vi "LIDAR V7 FPGA Main.vi"() -> ()   [LabVIEW 2013]
uses:
  Controls/FPGA Nain State.ctl
  Controls/Scan Format Typedaf.ctl
  <vilib>/Platform/TimedLoop/XDataNode/timing_clust.ctl
  <vilib>/Platform/TimedLoop/XDataNode/nitl_modes.ctl
  <vilib>/Platform/TimedLoop/XDataNode/wakeup.ctl
  Controls/Algorithm State.ctl
  <vilib>/rvi/Emulation/niFpgaSctlEmulationGetInTimedLoop.vi
  <vilib>/rvi/Emulation/niFpgaEmulationReportErrorSimple.vi
  <vilib>/rvi/Emulation/niFpgaGetClockAttributes.vi
  <vilib>/rvi/FIFO/Fifo_Resource/nirvififoEmulationReadFpgaImpl.vi
  <vilib>/rvi/DataTransferAndStorage/Container/Common/niFpgaContainerGetUniqueNameForEmu.vi
  <vilib>/rvi/eio/common/nirviEmuTemplateMethod_errors.vi
  <vilib>/rvi/Emulation/niFpgaCriticalErrorInLSC.vi
  <vilib>/rvi/Emulation/niFpgaProcessEmulError.vi
  LIDAR V2 Globals.vi
  <vilib>/rvi/FIFO/Fifo_Resource/nirvififoEmulationWriteFpgaImpl.vi
  <vilib>/rvi/IPIntegrationNode/IPINode_Utilities/niFpgaIPINodeSimCore.vi
  <vilib>/rvi/interface/RandomDataEmulation/nirviRandomDataFPGAFIFO.vi
  <vilib>/rvi/interface/RandomDataEmulation/niFpgaRandomDataHandleErrors.vi
  <vilib>/Platform/TimedLoop/XDataNode/XDataNode.xnode
  <vilib>/rvi/DataTransferAndStorage/Container/XNode/niFpgaContainer.xnode
  <vilib>/rvi/FIFO/Fifo_Resource/nirvififoEmulationRead.vi
  <vilib>/eio/EIONode/EIONode.xnode
  <vilib>/rvi/FIFO/Fifo_Resource/nirvififoEmulationWrite.vi
  <vilib>/rvi/XilinxIP/XIPIN_XNode/niFpgaXIPIN.xnode
  Frac Decimation test/FIR Compiler/FractionalDecimationV1.dll
  <vilib>/rvi/IPIntegrationNode/IPINode_Xnode/niFpgaIPINode.xnode
  <vilib>/rvi/FXPMathLib/FxpInterpret/XNode/nifxpmath_Interpret.xnode
  <vilib>/rvi/interface/RandomDataEmulation/nirviRandomDataFpgaReadWriteTemplate.vi
  <vilib>/Platform/TimedLoop/XDataNode/XDNodeRunTimeDep.lvlib
panel:
  out "AI 0":i16
  in  "MaxStartSample":u8
  in  "LedScanDebEn":bool
  in  "ActiveLedIndexDeb":u16
  in  "10thIndexDeb":u8
  in  "PulseUpClck":u16=3
  in  "PulseWaitClck":u16=40
  in  "AO Trig":bool
  in  "Devider":u8=3
  in  "PFI3":bool
  in  "PFI2":bool
  in  "User Command Commit":bool
  in  "User Command":u8
  out "User Command Idle":bool
  out "User Command Status":u8
  in  "User Data 0":u8
  in  "User Data 1":u8
  out "User Error":bool
  out "Configured?":bool
  in  "MemDebStart":u32
  in  "MemDebEnd":u32
  in  "ReadMemSel":bool
  in  "ReadMem":bool
  in  "NextLedEn":bool
  out "SimCoarsMaxIndex":u16
  out "SimFineMaxIndex":u16
  out "SimOut":i16
  out "SPI Idle":bool
  out "PLL Locked":bool
  in  "Clock":u8=1
  out "PLL Counter":i32
  in  "IO Module\\Apply Settings":bool
  out "LedAddress":u16
  in  "SingleCycle":bool
  in  "PulsePerLed":i16=199
  in  "ScanFormat":T1=enum."FullScanPerLed"
  in  "SamplingEnable":bool
  out "MainState":T2
  out "10thIndex":u8
  out "PulseIndex":i16
  in  "MemSel":bool
  in  "ActiveLedIndex":u16
  out "InitMem":bool
  out "PulseEnd":bool
  in  "SampPerPulse":u16=99
  out "IterReset":u16 format="%.0b"
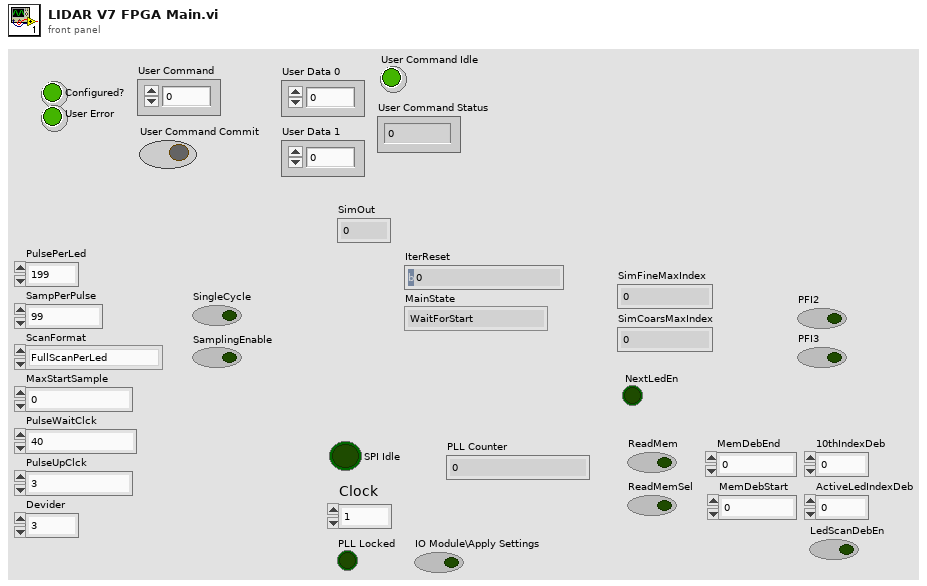
[diagram p1: front panel]
types:
  T1 = typedef "Scan Format Typedaf.ctl" = enum16{"1PulsePerLed", "FullScanPerLed"}
  T2 = typedef "FPGA Nain State.ctl" = enum16{"WaitForStart", "SetProcParams", "SelectActiveLed", "ActivatePulse", "WaitForPulseEnd", "WaitForAlgoStart", "SingleCycleEnd"}
  T3 = typedef "XDNodeRunTimeDep.lvlib/timing_clust.ctl" = cluster{"Expected End [f-1]":u64, "Actual End [f-1]":u64, "Finished Late? [f-1]":bool, "Expected End [i-1]":u64, "Actual End [i-1]":u64, "Finished Late? [i-1]":bool, "Expected Start [i]":u64, "Actual Start [i]":u64, "Expected Start [f]":u64, "Actual Start [f]":u64, "Source Name":string, "Structure Name":string, "Period":i64, "Deadline":i64, "Offset":i64, "Start":i64, "Priority":i32, "Timeout":i32, "Mode":T4, "Wakeup Reason":T5, "Error":errorcluster, "Source Type":string, "Secondary Source Type":string, "Global End Time":u64, "Global Start Time":u64, "Frame Duration":u64, "Iteration Duration":u64, "Assigned CPU":i32, "I/O Scan Engine Mode":u32}
  T4 = typedef "XDNodeRunTimeDep.lvlib/nitl_modes.ctl" = enum32{"No Change", "Process missed periods, maintain original phase", "Discard missed periods, maintain original phase", "Process missed periods, ignore original phase", "Discard missed periods, ignore original phase"}
  T5 = typedef "XDNodeRunTimeDep.lvlib/wakeup.ctl" = enum32{"Normal", "Aborted", "Asynchronous wakeup", "Timing source error", "Timed loop error", "Timeout"}
  T6 = typedef "Algorithm State.ctl" = enum16{"WaitForStart", "GetNextSignalElement", "WaitForNextSignalElem", "MultWithSinc", "CalcMax"}
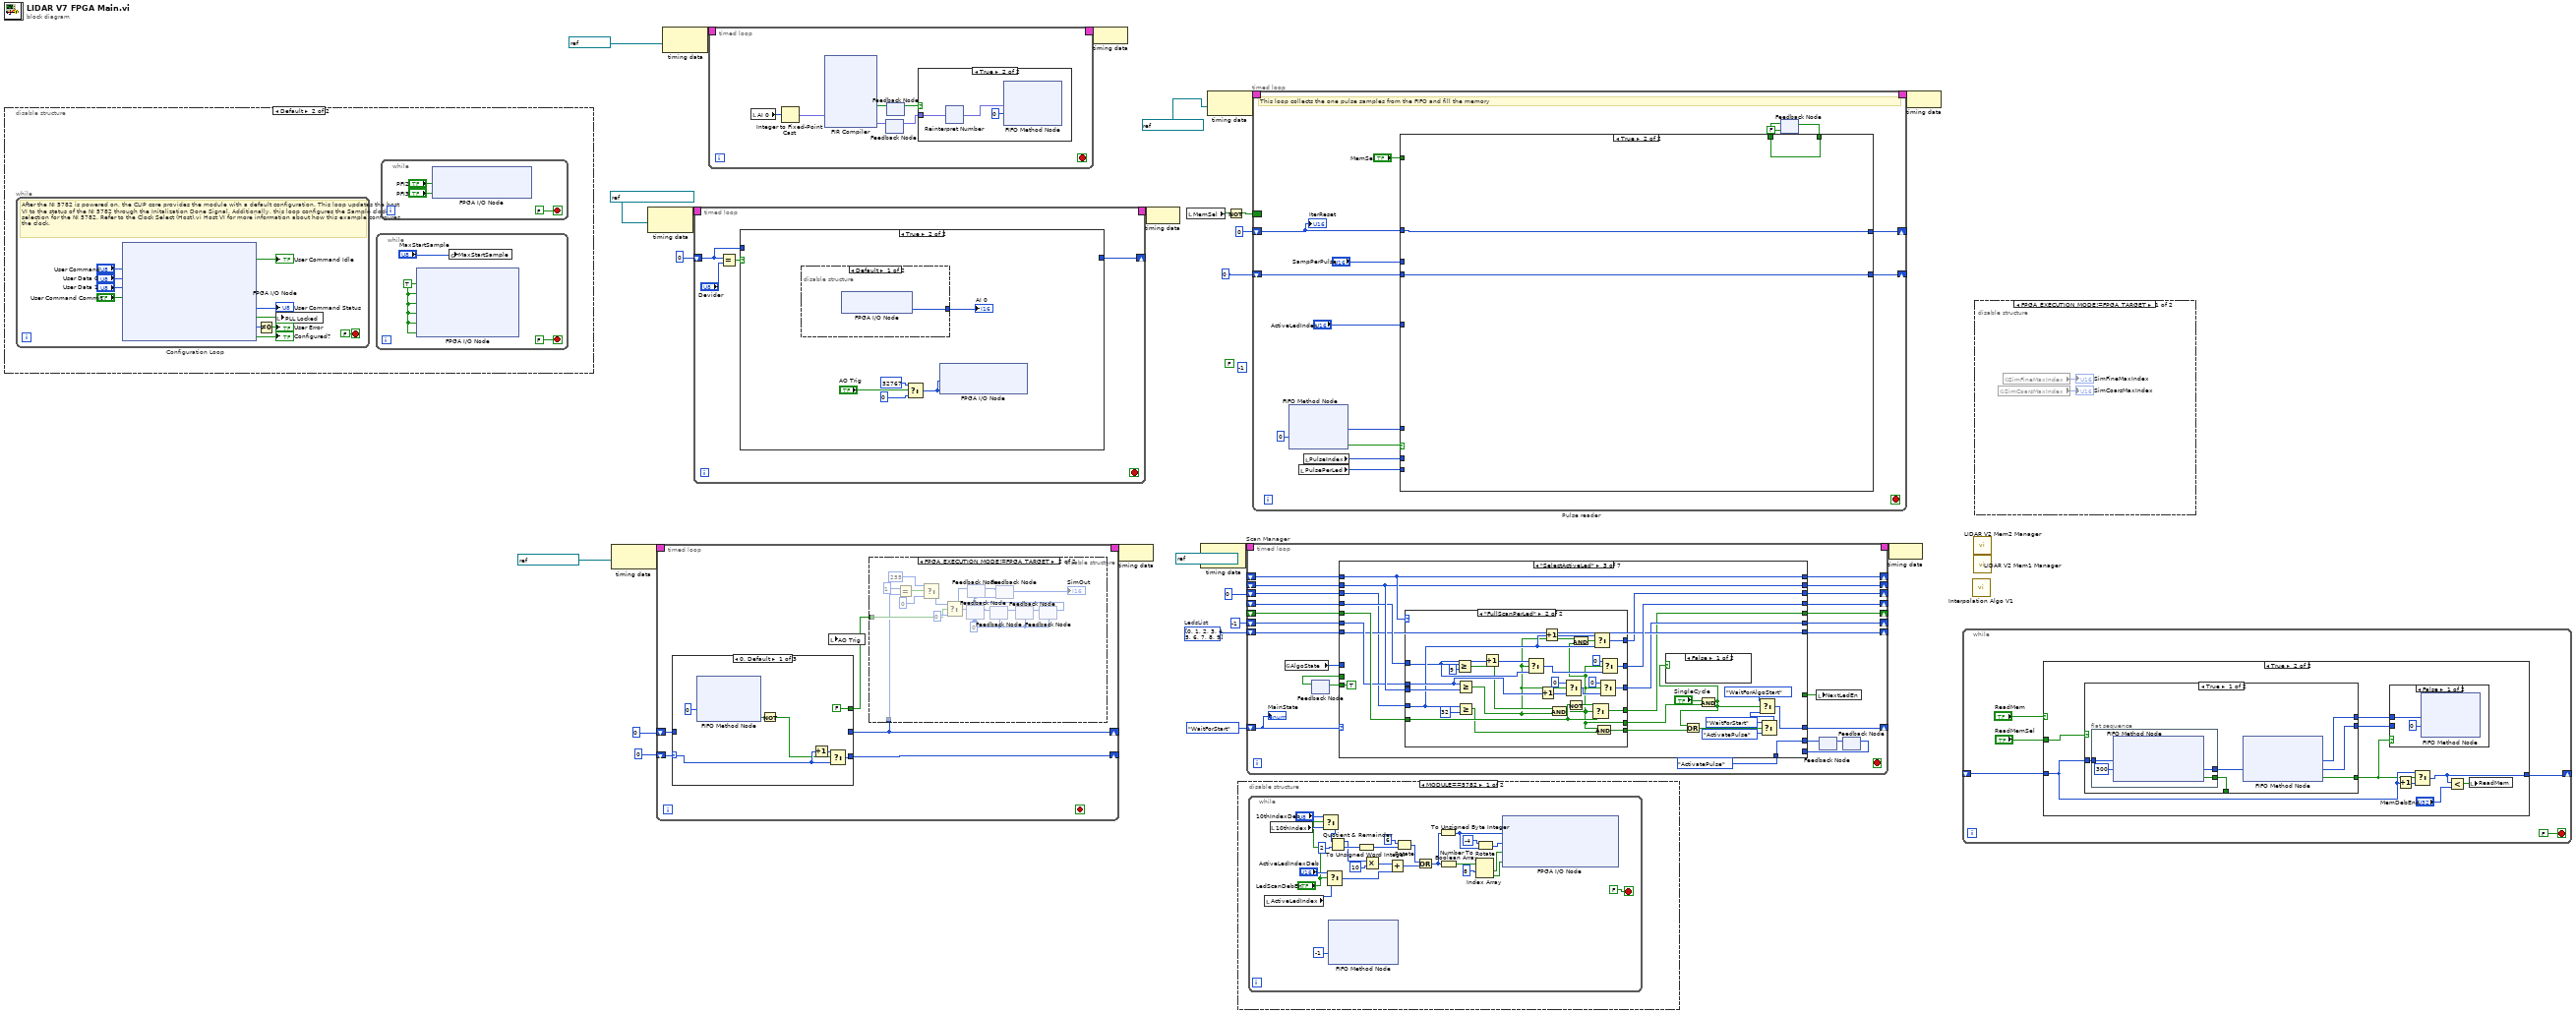
[diagram p0: block diagram]
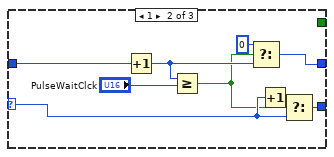
[diagram p4: hidden frame]
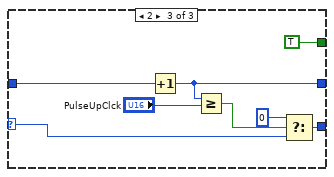
[diagram p5: hidden frame]
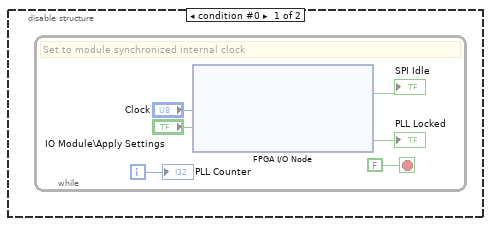
[diagram p7: hidden frame]
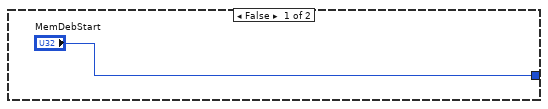
[diagram p8: hidden frame]
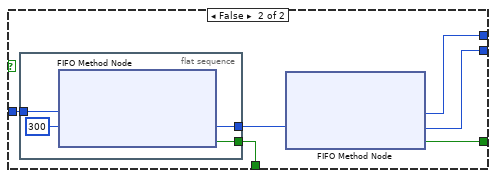
[diagram p10: hidden frame]
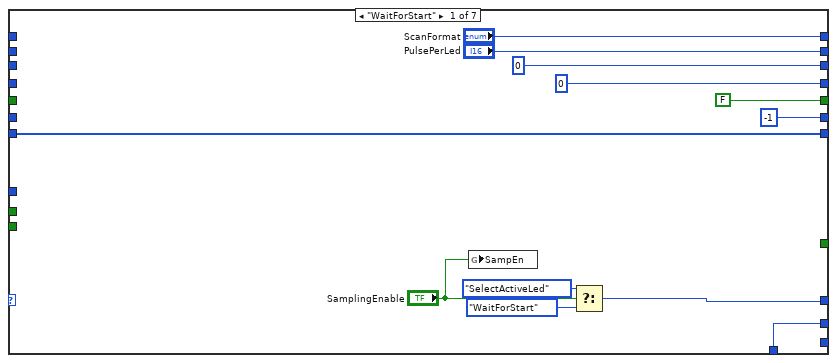
[diagram p12: hidden frame]
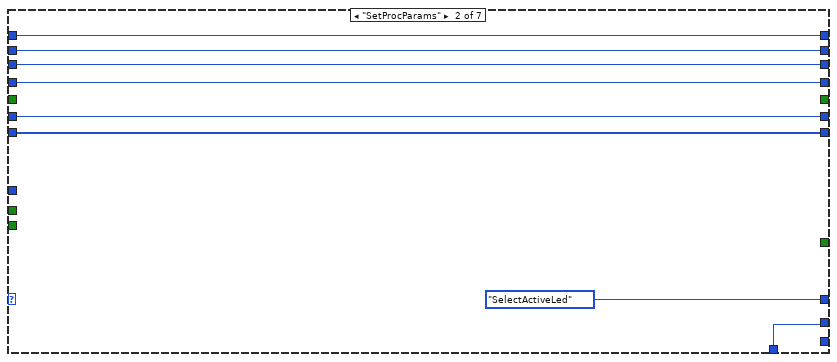
[diagram p13: hidden frame]
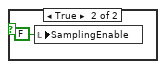
[diagram p14: hidden frame]
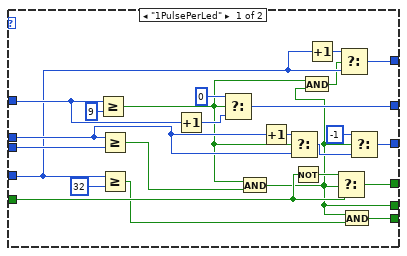
[diagram p15: hidden frame]
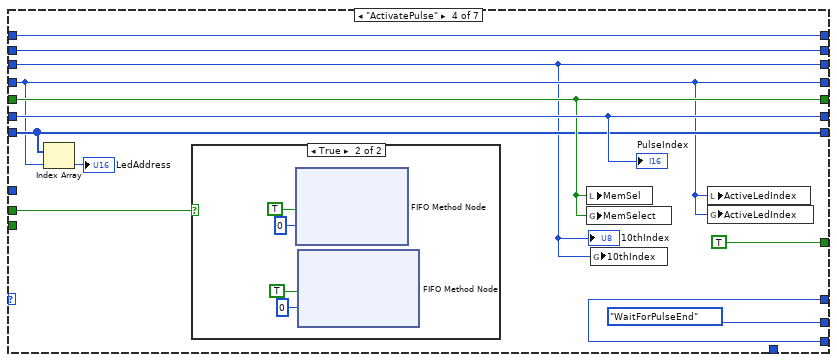
[diagram p16: hidden frame]
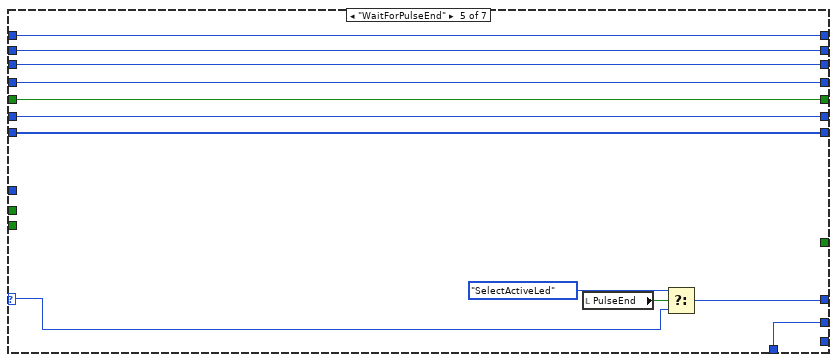
[diagram p18: hidden frame]
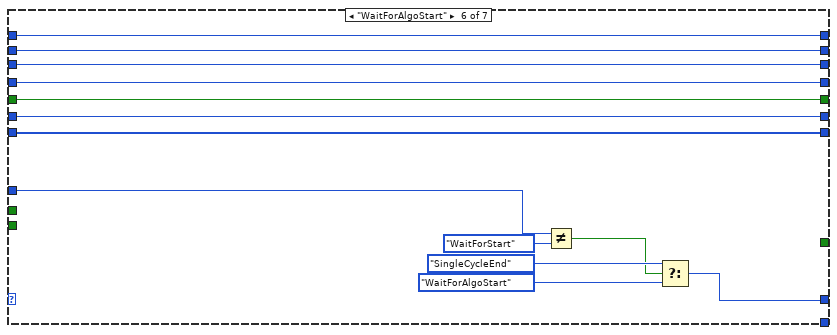
[diagram p19: hidden frame]
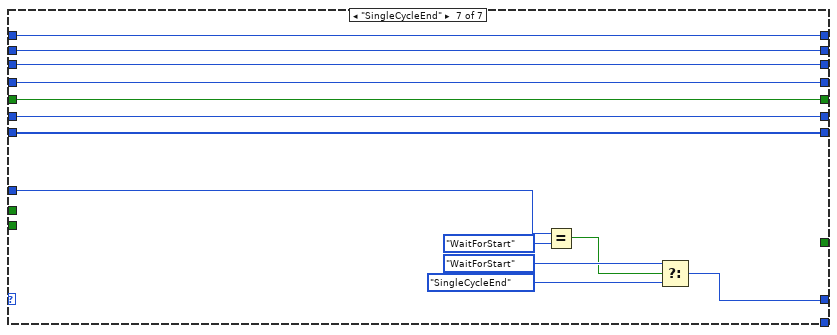
[diagram p20: hidden frame]
diagram:
  (unwired) FALSE
  w14 = u16[] [0, 1, 2, 3, 4, 5, 6, 7, 8, 9]  # LedsList
  (unwired) i16 -1 ("#Cycle")
  n1 = disable-structure shown="Default" {
    frame condition #0 {
      n2 = while {
        i -> [w29]
        stop <- FALSE stop-if-true
        # "Set to module synchronized internal clock"
        n3 = xnode "FPGA I/O Node"("IO Module\\Clock Select"="Clock", "IO Module\\Apply Settings"="IO Module\\Apply Settings") -> ("IO Module\\SPI Idle"=→"SPI Idle":bool, "IO Module\\PLL Locked"=→"PLL Locked":bool)  [unwired: 4 in, 4 out]
        "PLL Counter" <- w29
      }
    }
    frame condition #1 (active) {
      n4 = while "Configuration Loop" {
        stop <- FALSE stop-if-true
        # "After the NI 5782 is powered on, the CLIP core provides the module with a default configuration. This loop updates the host VI to the status of the NI 5782 through the Initalization Done Signal. Additionally, this loop configures the Sample clock selection for the NI 5782. Refer to the Clock Select (Host).vi Host VI for more information about how this example configures the clock."
        n5 = xnode "FPGA I/O Node"("IO Module\\User Command"="User Command", "IO Module\\User Data 0"="User Data 0", "IO Module\\User Data 1"="User Data 1", "IO Module\\User Command Commit"="User Command Commit") -> ("IO Module\\User Command Idle"=→"User Command Idle":bool, "IO Module\\User Command Status"=→"User Command Status":u8, "IO Module\\PLL Locked"=w36:bool, "IO Module\\User Error"=w40:u8, "IO Module\\Initialization Done"=→"Configured?":bool)  [unwired: 9 in, 9 out]
        n6 = Not Equal To 0?(x=w40) -> (x != 0?=→"User Error":bool)
        n7 = local write "PLL Locked"(w36) -> ()
      }
      n8 = while {
        stop <- FALSE stop-if-true
        w48 = TRUE ("IO Module\\DIO Port 0 WE")
        n9 = xnode "FPGA I/O Node"("IO Module\\DIO Port 0 WE"=w48, "IO Module\\DIO Port 1 WE"=w48, "IO Module\\PFI 0 WE"=w48, "IO Module\\PFI 1 WE"=w48, "IO Module\\PFI 2 WE"=w48, "IO Module\\PFI 3 WE"=w48) -> ()  [unwired: 6 in, 6 out]
        n10 = global write "LIDAR V2 Globals.vi" "MaxStartSample"("MaxStartSample") -> ()
      }
      n11 = while {
        stop <- FALSE stop-if-true
        n12 = xnode "FPGA I/O Node"("IO Module\\PFI 2 Wr Data"="PFI2", "IO Module\\PFI 3 Wr Data"="PFI3") -> ()  [unwired: 2 in, 2 out]
      }
    }
  }
  n13 = node-c288(refnum<k21> "100 MHz Clock" ("Source Name")) -> (w8:T3)
  n14 = node-c288(refnum<k21> "IO Module\\Data Clock" ("Source Name")) -> (w26:T3)
  n15 = timed-loop {
    timing: w8 -> [_]
    timing-out: [_] -> w7
    shift-right: [w53] -> _
    shift-left: i16 0 -> [w54]
    shift-right: [w51] -> _
    shift-left: u16 0 -> [w52]
    stop <- _ stop-if-true
    n16 = case shown="0, Default" w54 {
      selector: w54 -> [w76 w83 w89]
      tunnel: [w77 w84 w90] -> w53
      tunnel: w52 -> [_ w86 w94]
      tunnel: [_ w80 w93] -> w51
      tunnel: [FALSE _ TRUE] -> w50
      frame 0, Default {
        n17 = xnode ("FIFO Method Node")("Timeout"=0) -> ("Timed Out?"=w73:bool)  [unwired: 1 in, 2 out]
        n18 = Not(x=w73) -> (.not. x?=w71:bool)
        n19 = Increment(x=w76) -> (x+1=w75:i16)
        n20 = Select(t=w75, s=w71, f=w76) -> (s? t:f=w77:i16)
      }
      frame 1 {
        n21 = Increment(x=w86) -> (x+1=w81:u16)
        n22 = Greater Or Equal?(x=w81, y="PulseWaitClck") -> (x >= y?=w78:bool)
        n23 = Select(t=u16 0, s=w78, f=w81) -> (s? t:f=w80:u16)
        n24 = Increment(x=w83) -> (x+1=w82:i16)
        n25 = Select(t=w82, s=w78, f=w83) -> (s? t:f=w84:i16)
      }
      frame 2 {
        n26 = Increment(x=w94) -> (x+1=w93:u16)
        n27 = Greater Or Equal?(x=w93, y="PulseUpClck") -> (x >= y?=w91:bool)
        n28 = Select(t=i16 0, s=w91, f=w89) -> (s? t:f=w90:i16)
      }
    }
    n29 = local write "AO Trig"(w50) -> ()
    n30 = disable-structure shown="FPGA_EXECUTION_MODE!=FPGA_TARGET" {
      disable-tunnel: w50 -> [_ w62]
      disable-tunnel: w51 -> [_ w61]
      frame condition #0 (active) {
      }
      frame condition #1 {
        w65 = i16 0 ("IO Module\\AO 0")
        n31 = Equal?(x=u16 1, y=w61) -> (x = y?=w59:bool)
        n32 = Select(t=i16 255 ("IO Module\\AO 0"), s=w59, f=i16 0) -> (s? t:f=w60:i16)
        n33 = Select(t=w60, s=w62, f=i16 0 ("IO Module\\AO 0")) -> (s? t:f=w63:i16)
        n34 = feedback-in #1(w63) -> ()
        n35 = feedback #1(w65) -> (w70:i16)
        n36 = feedback #2(w65) -> (w66:i16)
        n37 = feedback #3(w65) -> (w69:i16)
        n38 = feedback-in #3(w70) -> ()
        n39 = feedback #4(w65) -> (→"SimOut":i16)
        n40 = feedback-in #4(w66) -> ()
        n41 = feedback #5(w65) -> (w68:i16)
        n42 = feedback-in #5(w69) -> ()
        n43 = feedback #6(w65) -> (w67:i16)
        n44 = feedback-in #2(w67) -> ()
        n45 = feedback-in #6(w68) -> ()
      }
    }
  }
  n46 = node-c288(refnum<k21> "300MHz" ("Source Name")) -> (w3:T3)
  n47 = timed-loop {
    timing: w26 -> [_]
    timing-out: [_] -> w25
    shift-right: [w97] -> _
    shift-left: u8 0 -> [w98]
    stop <- _ stop-if-true
    n48 = Equal?(x=w98, y="Devider") -> (x = y?=w99:bool)
    n49 = case shown="True" w99 {
      tunnel: w98 -> [w102 _]
      tunnel: [w101 _] -> w97
      frame False {
        n50 = Increment(x=w102) -> (x+1=w101:u8)
      }
      frame True {
        n51 = disable-structure shown="Default" {
          disable-tunnel: [w108 w109] -> w107
          frame condition #0 (active) {
            n52 = xnode "FPGA I/O Node"() -> ("IO Module\\AI 0"=w108:i16)  [unwired: 1 in, 1 out]
          }
          frame condition #1 {
            n53 = local read "SimOut"() -> (w109:i16)
          }
        }
        "AI 0" <- w107
        n54 = Select(t=i16 32767 ("IO Module\\AO 0"), s="AO Trig", f=i16 0 ("IO Module\\AO 0")) -> (s? t:f=w106:i16)
        n55 = xnode "FPGA I/O Node"("IO Module\\AO 0 N-1"=w106, "IO Module\\AO 0 N"=w106) -> ()  [unwired: 2 in, 2 out]
      }
    }
  }
  n56 = timed-loop {
    timing: w3 -> [_]
    timing-out: [_] -> w2
    stop <- _ stop-if-true
    n57 = local read "AI 0"() -> (w117:i16)
    n58 = Integer to Fixed-Point Cast(integer=w117) -> (fixed-point=w116:fxp<+/-,16,16>)  [unwired: 1 in]
    n59 = xnode ("FIR Compiler")("din"=w116) -> ("rdy"=w115:bool, "dout"=w114:fxp<+/-,33,33>)  [unwired: 1 out]
    n60 = feedback-in #7(w114) -> ()
    n61 = feedback #7() -> (w112:fxp<+/-,33,33>)  [unwired: 1 in]
    n62 = feedback-in #8(w115) -> ()
    n63 = feedback #8() -> (w113:bool)  [unwired: 1 in]
    n64 = case shown="True" w113 {
      tunnel: w112 -> [_ w166]
      frame False {
      }
      frame True {
        n65 = xnode "Reinterpret Number"("x"=w166) -> ("y"=w167:fxp<+/-,33,16>)
        n66 = xnode ("FIFO Method Node")("Element"=w167, "Timeout"=0) -> ()  [unwired: 1 in, 2 out]
      }
    }
  }
  n67 = node-c288(w2) -> ()
  n68 = node-c288(w7) -> ()
  n69 = node-c288(w25) -> ()
  n70 = local read "MemSel"() -> (w19:bool)
  n71 = node-c288(refnum<k21> "100 MHz Clock" ("Source Name")) -> (w22:T3)
  n72 = node-c288(refnum<k21> "100 MHz Clock" ("Source Name")) -> (w24:T3)
  n73 = Not(x=w19) -> (.not. x?=w18:bool)
  n74 = disable-structure shown="MODULE==5782" {
    frame condition #0 (active) {
      n75 = while {
        stop <- FALSE stop-if-true
        n76 = local read "ActiveLedIndex"() -> (w175:u16)
        n77 = local read "10thIndex"() -> (w177:u8)
        n78 = Select(t="10thIndexDeb", s="LedScanDebEn", f=w177) -> (s? t:f=w176:u8)
        n79 = Select(t="ActiveLedIndexDeb", s="LedScanDebEn", f=w175) -> (s? t:f=w174:u16)
        n80 = xnode ("FIFO Method Node")("Timeout"=-1) -> ()  [unwired: 1 in, 3 out]
        n81 = Quotient & Remainder(x=w176, y=u8 2) -> (x-y*floor(x/y)=w181:u8, floor(x/y)=w182:u8)
        n82 = To Unsigned Word Integer(number=w182) -> (unsigned 16bit integer=w189:u16)
        n83 = Multiply(x=w181, y=u8 10) -> (x*y=w180:u8)
        n84 = Add(x=w180, y=w174) -> (x+y=w195:u16)
        n85 = Rotate(1:w189, 2:u16 6 ("x")) -> (0:w196:u16)
        n86 = Or(x=w196, y=w195) -> (x .or. y?=w194:u16)
        n87 = To Unsigned Byte Integer(number=w194) -> (unsigned 8bit integer=w186:u8)
        n88 = Number To Boolean Array(number=w194) -> (Boolean array=w193:bool[])
        n89 = Index Array(array=w193, index #1=8 ("index")) -> (element #1=w191:bool, element #2=w190:bool)  [unwired: 1 in]
        n90 = Rotate(1:w186, 2:i16 -4 ("y")) -> (0:w184:u8)
        n91 = xnode "FPGA I/O Node"("IO Module\\DIO Port 0 Wr Data"=w186, "IO Module\\DIO Port 1 Wr Data"=w184, "IO Module\\PFI 0 Wr Data"=w191, "IO Module\\PFI 1 Wr Data"=w190) -> ()  [unwired: 4 in, 4 out]
      }
    }
    frame condition #1 {
    }
  }
  n92 = timed-loop "Scan Manager" {
    timing: w22 -> [_]
    timing-out: [_] -> w21
    shift-right: [w219] -> _
    shift-left: FPGA_Nain_State."WaitForStart" ("MainState") -> [w220]
    shift-right: [w218] -> _
    shift-left: _ -> [w216]
    shift-right: [w217] -> _
    shift-left: _ -> [w215]
    shift-right: [w208] -> _
    shift-left: u8 0 ("10thIndex") -> [w214]
    shift-right: [w198] -> _
    shift-left: _ -> [w213]
    shift-right: [w202] -> _
    shift-left: _ -> [w212]
    shift-right: [w211] -> _
    shift-left: i16 -1 -> [w201]
    shift-right: [w209] -> _
    shift-left: w14 -> [w210]
    stop <- _ stop-if-true
    n93 = global read "LIDAR V2 Globals.vi" "AlgoState"() -> (w197:T6)
    n94 = feedback #9() -> (w199:bool)  [unwired: 1 in]
    n95 = feedback #10() -> (w205:T2)  [unwired: 1 in]
    n96 = feedback #11() -> (w204:T2)  [unwired: 1 in]
    n97 = case shown="\"SelectActiveLed\"" w220 {
      selector: w220 -> [_ _ _ _ w336 _ _]
      tunnel: [w230 FPGA_Nain_State."SelectActiveLed" ("MainState") w244 w322 w335 w346 w359] -> w219
      tunnel: ["ScanFormat" w236 w263 w326 w342 w355 w368] -> w218
      tunnel: ["PulsePerLed" w235 w261 w325 w341 w354 w367] -> w217
      tunnel: w216 -> [_ w236 w263 w326 w342 w355 w368]
      tunnel: w215 -> [_ w235 w261 w325 w341 w354 w367]
      tunnel: [u8 0 ("10thIndex") w234 w252 w315 w340 w353 w366] -> w208
      tunnel: w214 -> [_ w234 w253 w315 w340 w353 w366]
      tunnel: [u16 0 ("ActiveLedIndex") w233 w258 w316 w339 w352 w365] -> w198
      tunnel: w213 -> [_ w233 w259 w316 w339 w352 w365]
      tunnel: [FALSE _ w255 w319 w338 w351 w364] -> w202
      tunnel: w212 -> [_ _ w262 w319 w338 w351 w364]
      tunnel: [i16 -1 ("t") w239 w256 w320 w333 w350 w363] -> w211
      tunnel: w201 -> [_ w239 w260 w320 w333 w350 w363]
      tunnel: w210 -> [w228 w238 w257 w317 w332 w349 w362]
      tunnel: [w228 w238 w257 w317 w332 w349 w362] -> w209
      tunnel: [_ _ _ TRUE ("SampEnable") _ _ _] -> w207
      tunnel: [w227 w237 w251 FPGA_Nain_State."WaitForPulseEnd" ("MainState") w331 _ _] -> w206
      tunnel: w204 -> [_ _ _ w322 _ _ _]
      tunnel: FPGA_Nain_State."ActivatePulse" ("MainState") -> [w227 w237 w251 _ w331 _ _]
      tunnel: [_ _ TRUE _ _ _ _] -> w200
      tunnel: w199 -> [_ _ _ w321 _ _ _]
      tunnel: w197 -> [_ _ _ _ _ w343 w357]
      frame "WaitForStart" {
        n98 = global write "LIDAR V2 Globals.vi" "SampEn"("SamplingEnable") -> ()
        n99 = Select(t=FPGA_Nain_State."SelectActiveLed" ("MainState"), s="SamplingEnable", f=FPGA_Nain_State."WaitForStart" ("MainState")) -> (s? t:f=w230:T2)
      }
      frame "SetProcParams" {
      }
      frame "SelectActiveLed" {
        n100 = case shown="\"FullScanPerLed\"" w263 {
          tunnel: w262 -> [w280 w310]
          tunnel: w253 -> [w273 w305]
          tunnel: w261 -> [w283 w312]
          tunnel: w259 -> [w286 w296]
          tunnel: w260 -> [w282 w311]
          tunnel: [w274 w292] -> w258
          tunnel: [w269 w294] -> w256
          tunnel: [w277 w308] -> w255
          tunnel: [w275 w306] -> w249
          tunnel: [w271 w303] -> w252
          tunnel: [w265 w289] -> w250
          frame "1PulsePerLed" {
            n101 = Greater Or Equal?(x=w286, y=u16 9) -> (x >= y?=w267:bool)
            n102 = Greater Or Equal?(x=w282, y=w283) -> (x >= y?=w278:bool)
            n103 = Greater Or Equal?(x=w273, y=u8 32) -> (x >= y?=w276:bool)
            n104 = Increment(x=w286) -> (x+1=w285:u16)
            n105 = Select(t=u16 0, s=w267, f=w285) -> (s? t:f=w274:u16)
            n106 = And(x=w267, y=w278) -> (x .and. y?=w265:bool)
            n107 = Increment(x=w282) -> (x+1=w281:i16)
            n108 = Select(t=w281, s=w267, f=w282) -> (s? t:f=w270:i16)
            n109 = Not(x=w280) -> (.not. x?=w279:bool)
            n110 = And(x=w267, y=w265) -> (x .and. y?=w266:bool)
            n111 = Increment(x=w273) -> (x+1=w272:u8)
            n112 = Select(t=w279, s=w265, f=w280) -> (s? t:f=w277:bool)
            n113 = Select(t=w272, s=w266, f=w273) -> (s? t:f=w271:u8)
            n114 = And(x=w265, y=w276) -> (x .and. y?=w275:bool)
            n115 = Select(t=i16 -1, s=w265, f=w270) -> (s? t:f=w269:i16)
          }
          frame "FullScanPerLed" {
            n116 = Greater Or Equal?(x=w296, y=u16 9) -> (x >= y?=w295:bool)
            n117 = Greater Or Equal?(x=w311, y=w312) -> (x >= y?=w290:bool)
            n118 = Greater Or Equal?(x=w305, y=u8 32) -> (x >= y?=w307:bool)
            n119 = Increment(x=w296) -> (x+1=w297:u16)
            n120 = Select(t=w297, s=w290, f=w296) -> (s? t:f=w293:u16)
            n121 = Increment(x=w311) -> (x+1=w299:i16)
            n122 = Increment(x=w305) -> (x+1=w304:u8)
            n123 = And(x=w295, y=w290) -> (x .and. y?=w289:bool)
            n124 = Select(t=i16 0, s=w290, f=w299) -> (s? t:f=w302:i16)
            n125 = Not(x=w310) -> (.not. x?=w309:bool)
            n126 = And(x=w290, y=w289) -> (x .and. y?=w300:bool)
            n127 = Select(t=w309, s=w289, f=w310) -> (s? t:f=w308:bool)
            n128 = Select(t=w304, s=w300, f=w305) -> (s? t:f=w303:u8)
            n129 = And(x=w289, y=w307) -> (x .and. y?=w306:bool)
            n130 = Select(t=i16 0, s=w289, f=w302) -> (s? t:f=w294:i16)
            n131 = Select(t=u16 0, s=w289, f=w293) -> (s? t:f=w292:u16)
          }
        }
        n132 = And(x="SingleCycle", y=w250) -> (x .and. y?=w241:bool)
        n133 = case shown="False" w241 {
          frame False {
          }
          frame True {
            n134 = local write "SamplingEnable"(FALSE ("SamplingEnable")) -> ()
          }
        }
        n135 = Or(x=w241, y=w249) -> (x .or. y?=w248:bool)
        n136 = Select(t=FPGA_Nain_State."WaitForStart" ("MainState"), s=w248, f=FPGA_Nain_State."ActivatePulse" ("MainState")) -> (s? t:f=w245:T2)
        n137 = Select(t=FPGA_Nain_State."WaitForAlgoStart" ("MainState"), s=w241, f=w245) -> (s? t:f=w244:T2)
      }
      frame "ActivatePulse" {
        n138 = Index Array(array=w317, index=w316) -> (element=→"LedAddress":u16)
        n139 = case shown="True" w321 {
          frame False {
          }
          frame True {
            n140 = xnode ("FIFO Method Node")("Element"=TRUE ("GenPulse"), "Timeout"=0) -> ()  [unwired: 1 in, 2 out]
            n141 = xnode ("FIFO Method Node")("Element"=TRUE ("GenPulse"), "Timeout"=0) -> ()  [unwired: 1 in, 2 out]
          }
        }
        n142 = local write "MemSel"(w319) -> ()
        n143 = global write "LIDAR V2 Globals.vi" "MemSelect"(w319) -> ()
        n144 = global write "LIDAR V2 Globals.vi" "10thIndex"(w315) -> ()
        n145 = local write "ActiveLedIndex"(w316) -> ()
        n146 = global write "LIDAR V2 Globals.vi" "ActiveLedIndex"(w316) -> ()
        "PulseIndex" <- w320
        "10thIndex" <- w315
      }
      frame "WaitForPulseEnd" {
        n147 = local read "PulseEnd"() -> (w337:bool)
        n148 = Select(t=FPGA_Nain_State."SelectActiveLed", s=w337, f=w336) -> (s? t:f=w335:T2)
      }
      frame "WaitForAlgoStart" {
        n149 = Not Equal?(x=w343, y=Algorithm_State."WaitForStart") -> (x != y?=w344:bool)
        n150 = Select(t=FPGA_Nain_State."SingleCycleEnd", s=w344, f=FPGA_Nain_State."WaitForAlgoStart" ("MainState")) -> (s? t:f=w346:T2)
      }
      frame "SingleCycleEnd" {
        n151 = Equal?(x=w357, y=Algorithm_State."WaitForStart") -> (x = y?=w356:bool)
        n152 = Select(t=FPGA_Nain_State."WaitForStart", s=w356, f=FPGA_Nain_State."SingleCycleEnd" ("MainState")) -> (s? t:f=w359:T2)
      }
    }
    n153 = feedback-in #9(w200) -> ()
    n154 = local write "NextLedEn"(w207) -> ()
    n155 = feedback-in #10(w206) -> ()
    n156 = feedback-in #11(w205) -> ()
    "MainState" <- w220
  }
  n157 = timed-loop "Pulse reader" {
    timing: w24 -> [_]
    timing-out: [_] -> w23
    shift-right: [w382] -> _
    shift-left: u16 0 -> [w380]
    border: w18 -> [_]
    shift-right: [w372] -> _
    shift-left: u16 0 -> [w371]
    stop <- _ stop-if-true
    # "This loop collects the one pulse samples from the FIFO and fill the memory"
    n158 = xnode ("FIFO Method Node")("Timeout"=0) -> ("Element"=w384:i16, "Timed Out?"=w383:bool)  [unwired: 1 in, 1 out]
    n159 = local read "PulsePerLed"() -> (w373:i16)
    n160 = local read "PulseIndex"() -> (w374:i16)
    n161 = feedback #12(FALSE) -> (w378:bool)
    n162 = case shown="True" w383 {
      tunnel: w384 -> [w436 _]
      tunnel: "ActiveLedIndex" -> [w389 _]
      tunnel: "SampPerPulse" -> [w435 _]
      tunnel: [w415 w447] -> w382
      tunnel: w380 -> [w437 w447]
      tunnel: [w394 w446] -> w379
      tunnel: w378 -> [w393 w446]
      tunnel: "MemSel" -> [w407 _]
      tunnel: w374 -> [w433 _]
      tunnel: w373 -> [w432 _]
      tunnel: [w387 w445] -> w372
      tunnel: w371 -> [w386 w445]
      frame False {
        w425 = u16 16384  # LastIterration
        w391 = u16 32768  # FirstIterration
        n163 = feedback #13() -> (w439:bool)
        n164 = feedback-in #13(w407) -> ()
        n165 = Greater Or Equal?(x=w386, y=w435) -> (x >= y?=w396:bool)
        "PulseEnd" <- w396
        n166 = Equal?(x=w433, y=w432) -> (x = y?=w434:bool)
        n167 = Not Equal?(x=w407, y=w439) -> (x != y?=w440:bool)
        n168 = Select(t=u16 0, s=w440, f=w437) -> (s? t:f=w392:u16)
        n169 = Multiply(x=w389, y=u16 100) -> (x*y=w430:u16)
        n170 = And(x=w389, y=u16 15) -> (x .and. y?=w421:u16)
        n171 = Add(x=w430, y=w386) -> (x+y=w429:u16)
        n172 = To Word Integer(number=w389) -> (16bit integer=w401:i16)
        n173 = Select(t=u16 0 ("x"), s=w393, f=w391) -> (s? t:f=w428:u16)
        n174 = Select(t=w425, s=w434, f=u16 0 ("x")) -> (s? t:f=w424:u16)
        n175 = Negate(x=w401) -> (-x=w397:i16)
        n176 = Or(x=w428, y=w429) -> (x .or. y?=w423:u16)
        n177 = Or(x=w423, y=w424) -> (x .or. y?=w418:u16)
        n178 = Rotate(1:w421, 2:i16 10 ("y")) -> (0:w419:u16)
        n179 = Or(x=w418, y=w419) -> (x .or. y?=w417:u16)
        n180 = Select(t=i16 2, s=w407, f=i16 0) -> (s? t:f=w403:i16)
        n181 = Select(t=i16 0, s=w396, f=i16 1) -> (s? t:f=w402:i16)
        n182 = Rotate(1:w392, 2:w397) -> (0:w398:u16)
        n183 = Logical Shift(y=w389, x=u16 1) -> (x << y=w412:u16)
        n184 = Join Numbers(hi=w436, lo=w417) -> ((hi.lo)=w427:u32)
        n185 = And(x=u16 1, y=w398) -> (x .and. y?=w400:u16)
        n186 = Or(x=w402, y=w403) -> (x .or. y?=w404:i16)
        n187 = Greater Than 0?(x=w400) -> (x > 0?=w395:bool)
        n188 = Or(x=w392, y=w412) -> (x .or. y?=w410:u16)
        n189 = case shown="1" w404 {
          tunnel: w427 -> [w441 w443 _]
          frame 1 {
            n190 = xnode ("FIFO Method Node")("Element"=w441, "Timeout"=0) -> ()  [unwired: 1 in, 2 out]
          }
          frame 3 {
            n191 = xnode ("FIFO Method Node")("Element"=w443, "Timeout"=0) -> ()  [unwired: 1 in, 2 out]
          }
          frame Default {
          }
        }
        n192 = Increment(x=w386) -> (x+1=w416:u16)
        n193 = Select(t=w386, s=w396, f=w416) -> (s? t:f=w388:u16)
        n194 = Select(t=w410, s=w396, f=w392) -> (s? t:f=w415:u16)
        n195 = Select(t=w395, s=w396, f=w393) -> (s? t:f=w394:bool)
        "InitMem" <- w394
        n196 = Select(t=u16 0, s="NextLedEn", f=w388) -> (s? t:f=w387:u16)
      }
      frame True {
      }
    }
    n197 = feedback-in #12(w379) -> ()
    "IterReset" <- w380
  }
  n198 = node-c288(w21) -> ()
  n199 = node-c288(w23) -> ()
  n200 = while {
    shift-right: [w452] -> _
    shift-left: _ -> [w451]
    stop <- FALSE stop-if-true
    n201 = case shown="True" "ReadMem" {
      tunnel: "ReadMemSel" -> [_ w459]
      tunnel: ["MemDebStart" w462] -> w452
      tunnel: w451 -> [_ w464]
      frame False {
      }
      frame True {
        n202 = case shown="True" w459 {
          tunnel: w464 -> [w471 w479]
          tunnel: [w470 w478] -> w456
          tunnel: [w469 w477] -> w458
          tunnel: [w468 w476] -> w457
          tunnel: [w467 w475] -> _
          frame True {
            n203 = flat-sequence {
              tunnel: w471 -> [w474]
              tunnel: [w473] -> w468
              tunnel: [w472] -> w467
              frame #0 {
                w473 = 300 ("Timeout")
                n204 = xnode ("FIFO Method Node")("Element"=w474, "Timeout"=w473) -> ("Timed Out?"=w472:bool)  [unwired: 1 in, 1 out]
              }
            }
            n205 = xnode ("FIFO Method Node")("Timeout"=w468) -> ("Element"=w469:u64, "Timed Out?"=w470:bool)  [unwired: 1 in, 1 out]
          }
          frame False {
            n206 = flat-sequence {
              tunnel: w479 -> [w482]
              tunnel: [w481] -> w476
              tunnel: [w480] -> w475
              frame #0 {
                w481 = 300 ("Timeout")
                n207 = xnode ("FIFO Method Node")("Element"=w482, "Timeout"=w481) -> ("Timed Out?"=w480:bool)  [unwired: 1 in, 1 out]
              }
            }
            n208 = xnode ("FIFO Method Node")("Timeout"=w476) -> ("Element"=w477:u64, "Timed Out?"=w478:bool)  [unwired: 1 in, 1 out]
          }
        }
        n209 = case shown="False" w456 {
          tunnel: w458 -> [w466 _]
          tunnel: w457 -> [_ _]
          frame False {
            n210 = xnode ("FIFO Method Node")("Element"=w466, "Timeout"=0) -> ()  [unwired: 1 in, 2 out]
          }
          frame True {
          }
        }
        n211 = Increment(x=w464) -> (x+1=w463:u32)
        n212 = Select(t=w464, s=w456, f=w463) -> (s? t:f=w462:u32)
        n213 = Less?(x=w462, y="MemDebEnd") -> (x < y?=w460:bool)
        n214 = local write "ReadMem"(w460) -> ()
      }
    }
  }
  n215 = call "Interpolation Algo V1.vi"() -> ()  [unwired: 10 in, 2 out]
  n216 = call "LIDAR V2 Mem2 Manager.vi"() -> ()  [unwired: 12 in]
  n217 = call "LIDAR V2 Mem1 Manager.vi"() -> ()  [unwired: 12 in]
  n218 = disable-structure shown="FPGA_EXECUTION_MODE!=FPGA_TARGET" {
    frame condition #0 {
      n219 = global read "LIDAR V2 Globals.vi" "SimCoarsMaxIndex"() -> (→"SimCoarsMaxIndex":u16)
      n220 = global read "LIDAR V2 Globals.vi" "SimFineMaxIndex"() -> (→"SimFineMaxIndex":u16)
    }
    frame condition #1 (active) {
    }
  }
